vi "get_buf2.vi"(4 "time GPS":timestamp caption="time" format="%<%.7X\n%x>T", 5 "Sync cluster":T1, 6 "Boolean":bool, 7 "Scope Cluster":T2={"instrument handle in"="", "ch list"="", "channels"="0,1,2,3"}) -> (0 "error out":errorcluster, 1 "Timing:GPS:Status":i32(ring) items=["Uninitialized", "Antenna Error", "No Useable Satellites", "One Useable Satellite", "Two Useable Satellites", "Three Useable Satellites", "No GPS Time", "PDOP Too High", "Unuseable Satellite", "Fix Rejected", "Self Survey Complete", "Self Survey Not Complete"], 2 "Device:Temperature":dbl)   [LabVIEW 2010]
uses:
  <instrlib>/niScope/Controls/niScope trigger source digital.ctl
  <instrlib>/niScope/Controls/niScope trigger slope.ctl
  <instrlib>/niScope/Controls/niScope vertical coupling.ctl
  <instrlib>/niScope/Acquire/Fetch/niScope Multi Fetch Binary 16.vi
  <instrlib>/niSync/niSync.llb/niSync Read Trigger Time Stamp (Multiple).vi
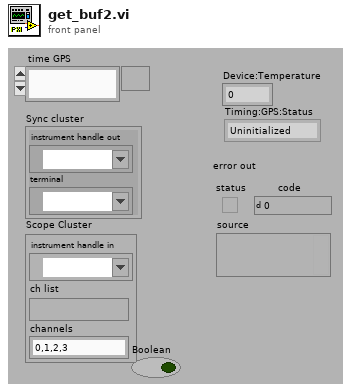
[diagram p1: front panel]
types:
  T1 = cluster{"instrument handle out":refnum<k15>, "terminal":tag}
  T2 = cluster{"instrument handle in":refnum<k15>, "ch list":string, "channels":string}
  T3 = typedef "niScope trigger source digital.ctl" = string
  T4 = cluster{"actualSamples":i32, "absoluteInitialX":dbl, "relativeInitialX":dbl, "xIncrement":dbl, "offset":dbl, "gain":dbl, "reserved1":dbl, "reserved2":dbl}[]
  T5 = typedef "niScope trigger slope.ctl" = i32
  T6 = typedef "niScope vertical coupling.ctl" = i32
  T7 = cluster{"input impedance":u32, enum16{"1/20", "1/5", "1", "6", "30"}, "vertical coupling":T6, "channels":string, "min sample rate":dbl, "reference position":dbl, i32, "trigger source":T3, "trigger slope":T5, dbl}
  T8 = cluster{"actualSamples":i32, "absoluteInitialX":dbl, "relativeInitialX":dbl, "xIncrement":dbl, "offset":dbl, "gain":dbl, "reserved1":dbl, "reserved2":dbl}
  T9 = cluster{cluster{"actualSamples":i32, "absoluteInitialX":dbl, "relativeInitialX":dbl, "xIncrement":dbl, "offset":dbl, "gain":dbl, "reserved1":dbl, "reserved2":dbl}[], "wfm":i16[][]}
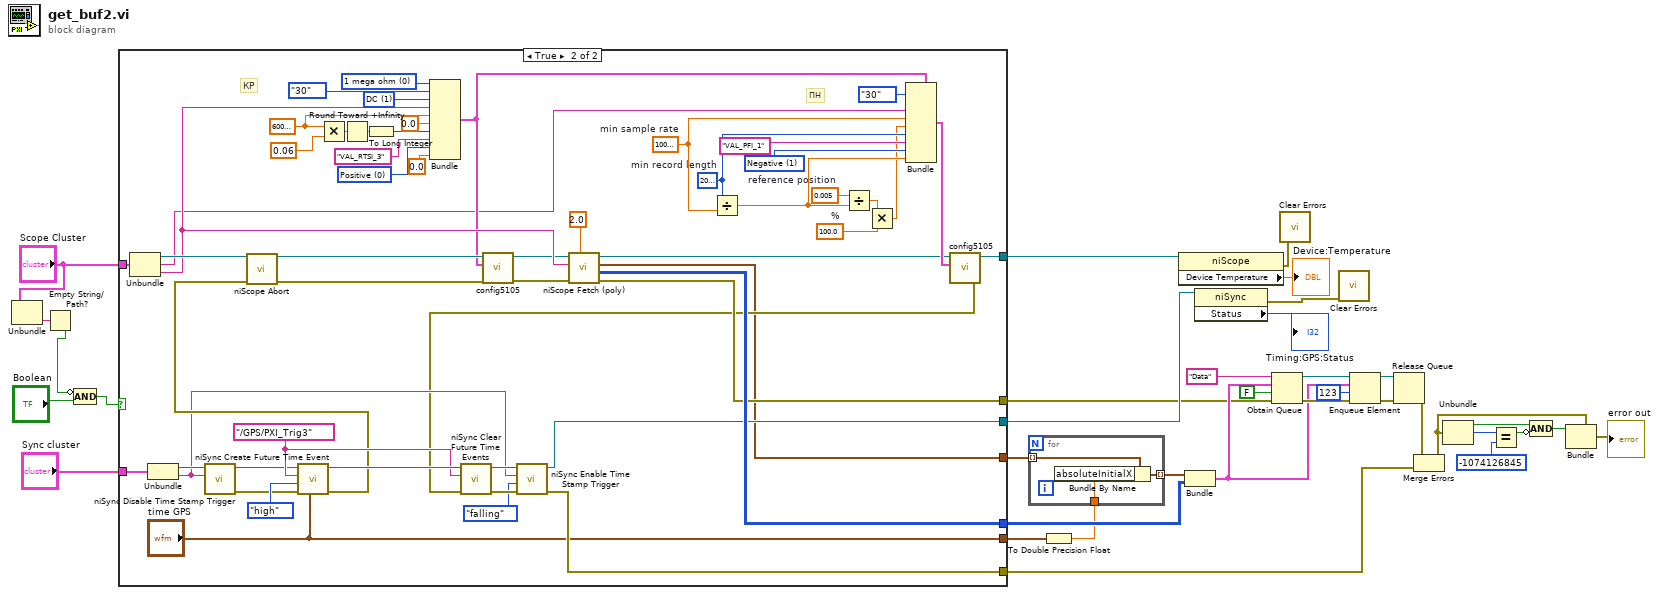
[diagram p0: block diagram]
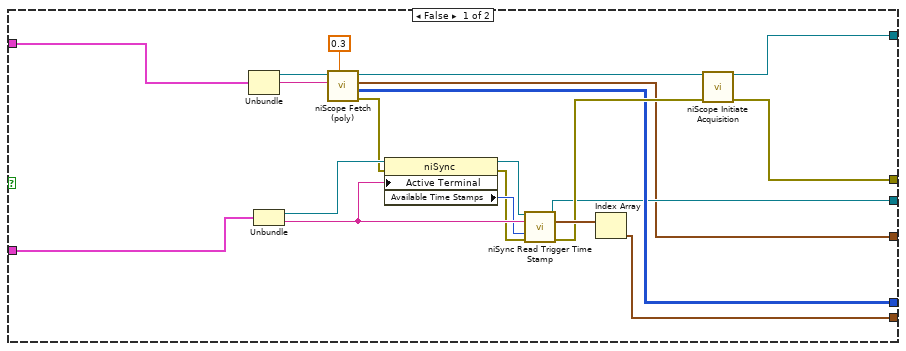
[diagram p2: hidden frame]
diagram:
  n1 = Unbundle("Scope Cluster") -> ("channels"=w8:string)  [unwired: 2 out]
  n2 = Empty String/Path?(string/path=w8) -> (empty?=w7:bool)
  n3 = Compound Arithmetic op=AND(invert w7, "Boolean") -> (w5:bool)
  n4 = case shown="True" w5 {
    tunnel: [w40 w109] -> w28
    tunnel: [w36 w58] -> w4
    tunnel: "Sync cluster" -> [w55 w103]
    tunnel: "Scope Cluster" -> [w47 w98]
    tunnel: [w41 w87] -> w12
    tunnel: [w39 w61] -> w17
    tunnel: [w38 w86] -> w16
    tunnel: [_ w85] -> w13
    tunnel: [w37 "time GPS"] -> w1
    frame False {
      n5 = Unbundle(w47) -> ("instrument handle in"=w42:refnum<k15>, "ch list"=w46:string)  [unwired: 1 out]
      n6 = Unbundle(w55) -> ("instrument handle out"=w54:refnum<k15>, "terminal"=w52:tag)
      n7 = call-poly <instrlib>:"niScope Fetch (poly).vi"("timeout"=0.3, "channels"=w46, "instrument handle"=w42) -> ("error out"=w49:errorcluster, "wfm"=w40:i16[][], "wfm info"=w36:T4, "instrument handle out"=w44:refnum<k15>)  [unwired: 5 in]
      n8 = property class="niSync"(reference=w54, error in=w49, "Active Terminal"=w52) -> (reference out=w53:refnum<k15>, error out=w48:errorcluster, "Available Time Stamps"=w51:i32)
      n9 = call-poly <instrlib>:"niSync Read Trigger Time Stamp.vi"("instrument handle"=w53, "terminal"=w52, "number of timestamps"=w51, "error in (no error)"=w48) -> ("instrument handle out"=w38:refnum<k15>, "time stamp out"=w50:timestamp[], "error out"=w43:errorcluster)  [unwired: 8 in, 1 out]
      n10 = Index Array(array=w50) -> (element=w37:timestamp)  [unwired: 1 in]
      n11 = call <instrlib>:"niScope Initiate Acquisition.vi"("instrument handle"=w44, "error in"=w43) -> ("instrument handle out"=w39:refnum<k15>, "error out"=w41:errorcluster)  [unwired: 12 in]
    }
    frame True {
      w93 = 100.0  # %
      w92 = 0.005  # reference position
      w69 = T5 1 items=["Positive", "Negative"] ("trigger slope")
      w65 = 2000000  # min record length
      w64 = 10000000.0  # min sample rate
      w106 = tag "/GPS/PXI_Trig3" ("terminal")
      w76 = T5 0 items=["Positive", "Negative"] ("trigger slope")
      w84 = u32 0 items=["1 mega ohm"=0, "50 ohms"=2] ("input impedance")
      w80 = 60000000.0 ("min sample rate")
      w82 = T6 1 items=["AC", "DC", "Ground"] ("vertical coupling")
      # "ПН"
      # "КР"
      n12 = Unbundle(w98) -> ("instrument handle in"=w96:refnum<k15>, "ch list"=w66:string, "channels"=w81:string)
      n13 = Unbundle(w103) -> ("instrument handle out"=w102:refnum<k15>, "terminal"=w88:tag)
      n14 = call <instrlib>:"niSync Disable Time Stamp Trigger.vi"("terminal"=w88, "instrument handle"=w102) -> ("error out"=w99:errorcluster, "instrument handle out"=w100:refnum<k15>)  [unwired: 7 in]
      n15 = call <instrlib>:"niSync Create Future Time Event.vi"("time"="time GPS", "error in (no error)"=w99, "output level"=enum32{"low", "high"}."high", "terminal"=w106, "instrument handle"=w100) -> ("error out"=w95:errorcluster, "instrument handle out"=w107:refnum<k15>)  [unwired: 4 in]
      n16 = call <instrlib>:"niScope Abort.vi"("instrument handle"=w96, "error in"=w95) -> ("instrument handle out"=w71:refnum<k15>, "error out"=w72:errorcluster)  [unwired: 12 in]
      n17 = Multiply(x=w80, y=0.06 ("x")) -> (x*y=w108:dbl)
      n18 = Round Toward +Infinity(x=w108) -> (ceil(x): smallest int >= x=w104:dbl)
      n19 = To Long Integer(number=w104) -> (32bit integer=w78:i32)
      n20 = Bundle("input impedance"=w84, enum16{"1/20", "1/5", "1", "6", "30"}."30", "vertical coupling"=w82, "channels"=w81, "min sample rate"=w80, "reference position"=0.0, w78, "trigger source"=T3 "VAL_RTSI_3", "trigger slope"=w76, 0.0) -> (w70:T7)  [unwired: 1 in]
      n21 = call "config5105.vi"("error in"=w72, "Cluster"=w70, "instrument handle"=w71) -> ("error out"=w73:errorcluster, "instrument handle out"=w74:refnum<k15>)  [unwired: 3 in]
      n22 = call-poly <instrlib>:"niScope Fetch (poly).vi"("timeout"=2.0 ("x"), "error in"=w73, "channels"=w81, "instrument handle"=w74) -> ("error out"=w87:errorcluster, "wfm"=w109:i16[][], "wfm info"=w58:T4, "instrument handle out"=w59:refnum<k15>)  [unwired: 4 in]
      n23 = Divide(x=w65, y=w64) -> (x/y=w67:dbl)
      n24 = Divide(x=w92, y=w67) -> (x/y=w94:dbl)
      n25 = Multiply(x=w94, y=w93) -> (x*y=w63:dbl)
      n26 = Bundle(cluster=w70, enum16{"1/20", "1/5", "1", "6", "30"}."30", "channels"=w66, "min sample rate"=w64, "reference position"=w63, w65, "trigger source"=T3 "VAL_PFI_1", "trigger slope"=w69, w67) -> (w60:T7)  [unwired: 2 in]
      n27 = call "config5105.vi"("Cluster"=w60, "instrument handle"=w59) -> ("error out"=w62:errorcluster, "instrument handle out"=w61:refnum<k15>)  [unwired: 4 in]
      n28 = call <instrlib>:"niSync Clear Future Time Events.vi"("error in (no error)"=w62, "terminal"=w106, "instrument handle"=w107) -> ("error out"=w91:errorcluster, "instrument handle out"=w90:refnum<k15>)  [unwired: 6 in]
      n29 = call <instrlib>:"niSync Enable Time Stamp Trigger.vi"("error in (no error)"=w91, "active edge"=enum32{"rising", "falling", "any"}."falling", "terminal"=w88, "instrument handle"=w90) -> ("error out"=w85:errorcluster, "instrument handle out"=w86:refnum<k15>)  [unwired: 5 in]
    }
  }
  n30 = To Double Precision Float(number=w1) -> (double precision float=w2:dbl)
  n31 = for {
    tunnel: w4 -> [w112] mode=indexing
    tunnel: [w111] -> w3 mode=indexing
    tunnel: w2 -> [w110]
    n32 = Bundle By Name(cluster=w112, "absoluteInitialX"=w110) -> (w111:T8)
  }
  n33 = property class="niScope"(reference=w17) -> (error out=w11:errorcluster, "Device Temperature"=→"Device:Temperature":dbl)  [unwired: 1 in, 1 out]
  n34 = Bundle(w3, "wfm"=w28) -> (w26:T9)  [unwired: 1 in]
  n35 = property class="niSync"(reference=w16) -> (error out=w10:errorcluster, "Status"=→"Timing:GPS:Status":i32)  [unwired: 1 in, 1 out]
  n36 = Obtain Queue(name (unnamed)="Data", element data type=w26, create if not found? (T)=FALSE, error in (no error)=w12) -> (queue out=w32:refnum<queue>, error out=w30:errorcluster)  [unwired: 1 in, 1 out]
  n37 = call <vilib>:"Clear Errors.vi"("error in (no error)"=w11) -> ()  [unwired: 6 in, 1 out]
  n38 = call <vilib>:"Clear Errors.vi"("error in (no error)"=w10) -> ()  [unwired: 6 in, 1 out]
  n39 = Enqueue Element(queue=w32, element=w26, timeout in ms (-1)=123, error in (no error)=w30) -> (queue out=w31:refnum<queue>, error out=w29:errorcluster)  [unwired: 1 out]
  n40 = Release Queue(queue=w31, error in (no error)=w29) -> (error out=w20:errorcluster)  [unwired: 1 in, 2 out]
  n41 = Merge Errors(w20, w13) -> (w19:errorcluster)
  n42 = Unbundle(w19) -> ("status"=w21:bool, "code"=w25:i32)  [unwired: 1 out]
  n43 = Equal?(x=w25, y=-1074126845) -> (x = y?=w23:bool)
  n44 = Compound Arithmetic op=AND(w21, invert w23) -> (w22:bool)
  n45 = Bundle(cluster=w19, "status"=w22) -> (→"error out":errorcluster)  [unwired: 2 in]
